vi "Configure Digital Input Baseband Frequency Offset.vi"(8 "error in (no error)":errorcluster, 10 "Baseband Frequency Offset (0.00000000E+000 Hz)":dbl format="%_6e", 11 "VISA resource name":refnum<visa-resource-name>) -> (0 "error out":errorcluster, 3 "VISA resource name out":refnum<visa-resource-name>)   [LabVIEW 2018, in "Agilent PSG MXG Series.lvlib"]
doc: "Configures the digital input baseband.\n\n<b>Note:</b>\nIt is applicable for N5172B/82B with <b>Option 004</b> only."
uses:
  Agilent PSG MXG Series.lvlib
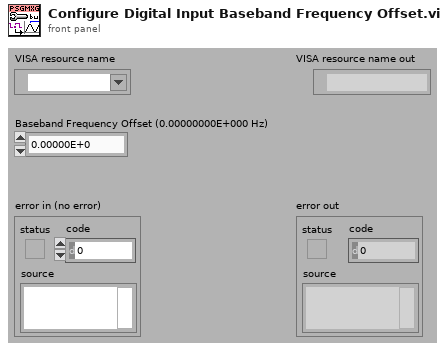
[diagram p1: front panel]
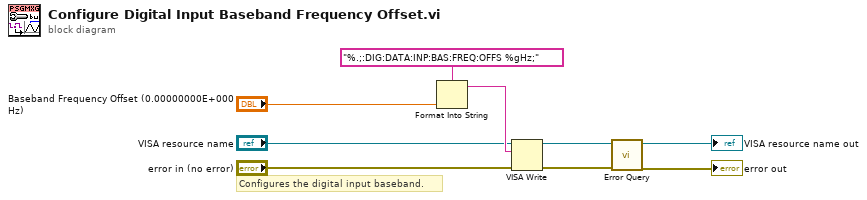
[diagram p0: block diagram]
diagram:
  # "Configures the digital input baseband."
  n1 = Format Into String(format string="%.;:DIG:DATA:INP:BAS:FREQ:OFFS %gHz;", "Baseband Frequency Offset (0.00000000E+000 Hz)") -> (resulting string=w7:string)  [unwired: 2 in, 1 out]
  n2 = VISA Write(VISA resource name="VISA resource name", write buffer=w7, error in (no error)="error in (no error)") -> (VISA resource name out=w4:refnum<visa-resource-name>, error out=w3:errorcluster)  [unwired: 1 out]
  n3 = call "Error Query.vi"("error in (no error)"=w3, "VISA resource name"=w4) -> ("error out"=→"error out":errorcluster, "VISA resource name out"=→"VISA resource name out":refnum<visa-resource-name>)  [unwired: 6 in, 2 out]
